vi "XML_String.vi"(1 "variable":i32, 2 "variable name":string="test") -> (0 "xml string":string)   [LabVIEW 2012]
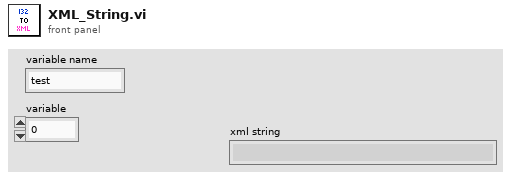
[diagram p1: front panel]
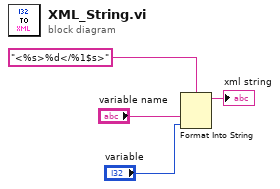
[diagram p0: block diagram]
diagram:
  n1 = Format Into String(format string="<%s>%d</%1$s>" ("format string (<%s>%d</%1$s>)"), "variable name", "variable") -> (resulting string=→"xml string":string)  [unwired: 2 in, 1 out]
